vi "Main.vi"(11 "Module Admin":refnum<class "Delacor_lib_QMH_Module Admin.lvclass">) -> ()   [LabVIEW 2023, in "Analog Input.lvlib"]
doc: "This template is based off of the Queued Message Handler design pattern and the Queued Message Handler project template that ships with LabVIEW.\n\nThe main difference is that the queue is private to this module and communication between modules is performed via Broadcast and Request events.\n\nRequest events are wrapped in public API methods and are handled in the Event Handling Loop (EHL) of this VI. Any module can register for Broadcast events sent by this module. The EHL generates messages based on user interface actions.\n\nThe Message Handling Loop (MHL) processes messages generated by the EHL, or by other messages. The messages are string values, so new messages can be added easily to the Message Cases case structure in the MHL. Each message cluster can also provide an optional value for Message Data, which is a variant that can be converted to whatever message-specific data is required.\n_____\nBased on DQMH Dev Tools: Project Template 7.1.1.1528."
uses:
  Analog Input.lvlib
  <vilib>/Delacor/Delacor QMH/Libraries/Module Admin_class/Delacor_lib_QMH_Module Admin.lvclass
  Module Data--cluster.ctl
  <vilib>/myRIO/Instrument Drivers/Onboard IO/AI/typedefs/AI Reference.ctl
  <vilib>/myRIO/Common/Instrument Driver Framework/Utilities/typedefs/myRIO Generic Hardware Reference.ctl
  <vilib>/myRIO/Common/Instrument Driver Framework/Utilities/typedefs/Hardware Version Enum.ctl
  <vilib>/myRIO/Common/Instrument Driver Framework/Utilities/typedefs/myRIO v1.0 Reference.ctl
  <vilib>/myRIO/Common/Instrument Driver Framework/Utilities/typedefs/Generic FPGA Reference.ctl
  <vilib>/myRIO/Common/Instrument Driver Framework/myRIO v1.0/AI/typedefs/AI Channels List.ctl
  <vilib>/myRIO/Common/Instrument Driver Framework/myRIO v1.0/AI/typedefs/AI Channels Enum.ctl
  <vilib>/myRIO/Common/Instrument Driver Framework/Utilities/typedefs/Analog Scaling Constants List.ctl
  <vilib>/myRIO/Common/Instrument Driver Framework/Utilities/typedefs/Analog Scaling Constants.ctl
  Stop Argument--cluster.ctl
  <vilib>/Delacor/Delacor QMH/Libraries/Message Queue_class/Delacor_lib_QMH_Message Queue.lvclass/Delacor_lib_QMH_Message Queue.ctl
  <vilib>/Delacor/Delacor QMH/Libraries/Module Admin_class/Delacor_lib_QMH_Module Admin.lvclass/Delacor_lib_QMH_Module Admin.ctl
  <vilib>/userDefined/High Color/nirio_resource_hc.ctl
  <vilib>/Delacor/Delacor QMH/Libraries/Message Queue_class/Delacor_lib_QMH_Enqueue Message (Single).vi
  <vilib>/Delacor/Delacor QMH/Libraries/Module Admin_class/Delacor_lib_QMH_Get External Launch.vi
  <vilib>/myRIO/Common/Instrument Driver Framework/myRIO v1.0/AI/vis/myRIO v1.1 Open AI.vi
  <vilib>/myRIO/Common/Instrument Driver Framework/Utilities/vis/Validate Channels.vi
  <vilib>/myRIO/Common/Instrument Driver Framework/myRIO v1.0/AI/vis/myRIO v1.0 Reserve AI.vi
  <vilib>/myRIO/Common/Instrument Driver Framework/myRIO v1.0/AI/vis/myRIO v1.0 Close AI.vi
  <vilib>/myRIO/Common/Instrument Driver Framework/myRIO v1.0/AI/vis/myRIO v1.0 Build MUX Configuration AI.vi
  <vilib>/myRIO/Common/Instrument Driver Framework/myRIO v1.0/Resource Manager/vis/myRIO v1.0 Reserve Channel List.vi
  <vilib>/myRIO/Common/Instrument Driver Framework/myRIO v1.0/AI/vis/myRIO v1.0 Unreserve AI.vi
  <vilib>/myRIO/Common/Instrument Driver Framework/myRIO v1.0/Resource Manager/vis/myRIO v1.0 Reserve Channel.vi
  <vilib>/myRIO/Common/Instrument Driver Framework/myRIO v1.0/Resource Manager/vis/myRIO v1.0 Unreserve Channel.vi
  <vilib>/myRIO/Common/Instrument Driver Framework/myRIO v1.0/Resource Manager/vis/myRIO v1.0 Unreserve Channel List.vi
  <vilib>/myRIO/Common/Instrument Driver Framework/myRIO v1.0/Resource Manager/vis/myRIO v1.0 Build Mutex Name.vi
  <vilib>/Utility/VariantDataType/GetNumericInfo.vi
  <vilib>/myRIO/Common/Instrument Driver Framework/myRIO v1.0/myRIO v1.1 Open.vi
  <vilib>/myRIO/Common/Instrument Driver Framework/myRIO v1.0/AI/vis/myRIO v1.0 Get Scaling Constants AI.vi
  <vilib>/myRIO/Common/Instrument Driver Framework/Utilities/vis/IO Manager.vi
  <vilib>/myRIO/Common/Instrument Driver Framework/Utilities/vis/Configuration Manager.vi
  <vilib>/myRIO/Common/Instrument Driver Framework/myRIO v1.0/myRIO v1.0 Close.vi
  <vilib>/myRIO/Common/Instrument Driver Framework/myRIO v1.0/AI/vis/myRIO v1.0 Read AI.vi
  <vilib>/myRIO/Instrument Drivers/Onboard IO/AI/vis/myRIO AI Open.xnode
  <vilib>/Delacor/Delacor QMH/Libraries/Message Queue_class/Delacor_lib_QMH_Message Queue.lvclass
  <vilib>/myRIO/Instrument Drivers/Onboard IO/AI/AI.lvlib
panel:
  out "error out":errorcluster
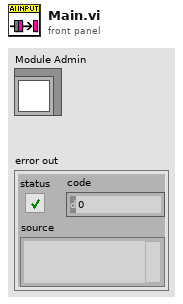
[diagram p1: front panel]
types:
  T1 = typedef "Analog Input.lvlib/Request Events--cluster.ctl" = cluster{"Stop Module":refnum<user-event>, "Show Panel":refnum<user-event>, "Hide Panel":refnum<user-event>, "Get Module Execution Status":refnum<user-event>, "Show Diagram":refnum<user-event>, "Private.Open Connection":refnum<user-event>, "Read Analog":refnum<user-event>}
  T2 = typedef "Analog Input.lvlib/Module Data--cluster.ctl" = cluster{"Status":string, "AI Reference":T3}
  T3 = typedef "AI.lvlib/AI Reference.ctl" = cluster{"myRIO Reference":T4, "AI Channels List":T8, "AI Scaling Constants List":T10}
  T4 = typedef "myRIO Generic Hardware Reference.ctl" = cluster{"myRIO Model":T5, "myRIO Hardware Reference":T6}
  T5 = typedef "Hardware Version Enum.ctl" = enum16{"Unknown", "myRIO-1900", "myRIO-1950", "roboRIO", "NI ELVIS RIO CM", "ELVIS III"}
  T6 = typedef "myRIO v1.0 Reference.ctl" = cluster{"Generic FPGA Reference":T7, "Allow multiple opens":bool}
  T7 = typedef "Generic FPGA Reference.ctl" = refnum<k20>
  T8 = typedef "AI Channels List.ctl" = T9[]
  T9 = typedef "AI Channels Enum.ctl" = enum16{"Not Connected", "AudioIn/Left", "AudioIn/Right", "C/AI0", "C/AI1", "A/AI0", "A/AI1", "A/AI2", "A/AI3", "A/AI4", "A/AI5", "A/AI6", "A/AI7", "B/AI0", "B/AI1", "B/AI2", "B/AI3", "B/AI4", "B/AI5", "B/AI6", "B/AI7", "AI/AI0", "AI/AI1", "AI/AI2", "AI/AI3", "A/AI0 (DIFF)", "A/AI1 (DIFF)", "A/AI2 (DIFF)", "A/AI3 (DIFF)", "B/AI0 (DIFF)", "B/AI1 (DIFF)", "B/AI2 (DIFF)", "B/AI3 (DIFF)"}
  T10 = typedef "Analog Scaling Constants List.ctl" = T11[]
  T11 = typedef "Analog Scaling Constants.ctl" = cluster{"LSB Weight (Volts)":dbl, "Offset (Volts)":dbl, "Signed?":bool}
  T12 = enum32{"invalid lock state", "Not Locked", "Locked (No Password)", "Password-protected"}
  T13 = typedef "Analog Input.lvlib/Stop Argument--cluster.ctl" = cluster{"Origin":string, "Exit via Stop Module Req?":bool, "Wait for Module to stop?":bool}
  T14 = typedef "nirio_resource_hc.ctl" = tag
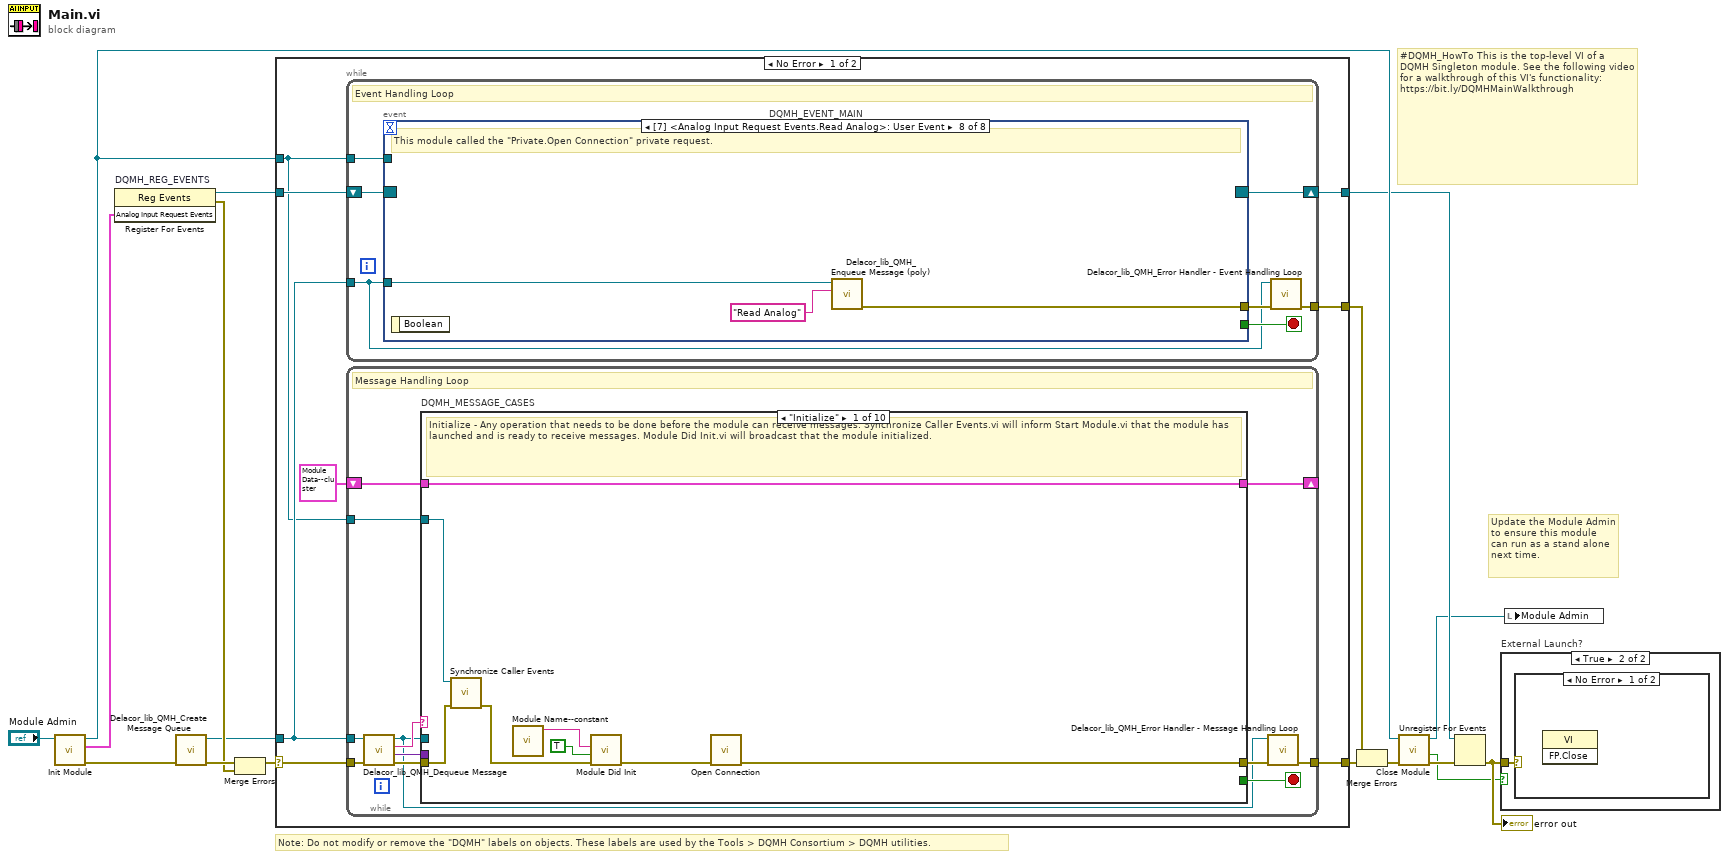
[diagram p0: block diagram]
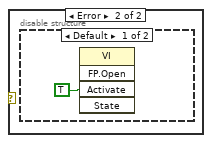
[diagram p3: hidden frame]
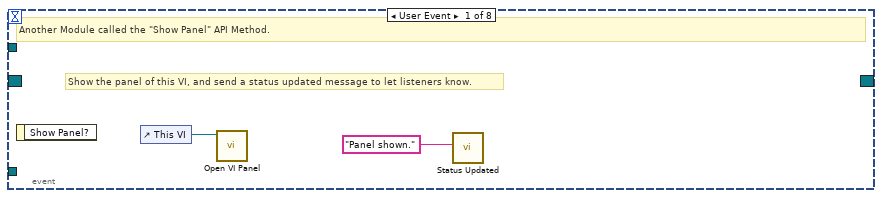
[diagram p5: hidden frame]
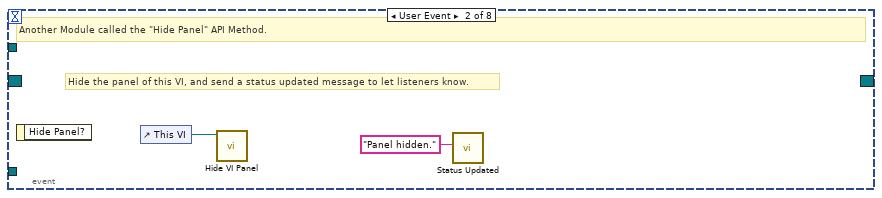
[diagram p6: hidden frame]
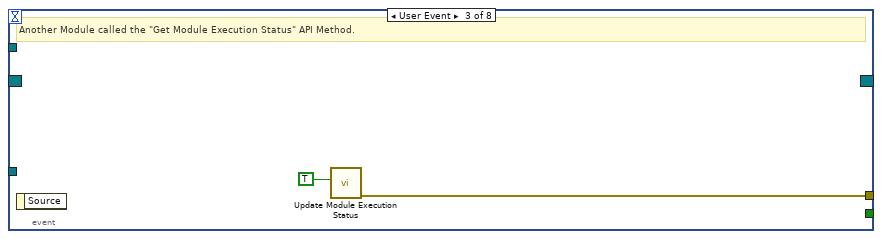
[diagram p7: hidden frame]
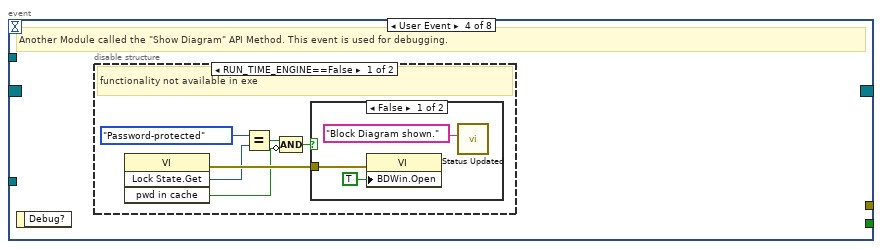
[diagram p8: hidden frame]
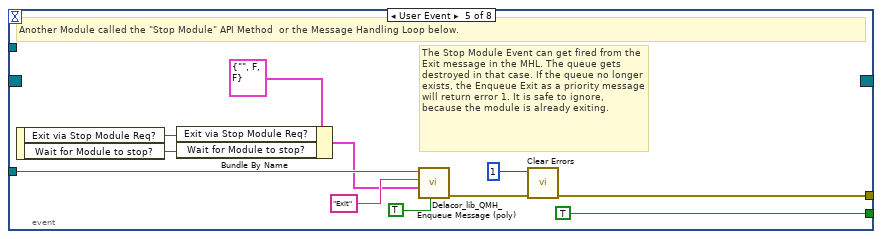
[diagram p11: hidden frame]
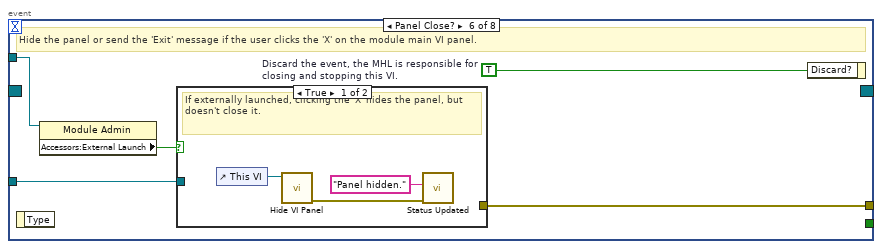
[diagram p12: hidden frame]
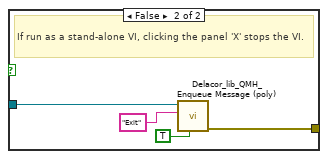
[diagram p13: hidden frame]
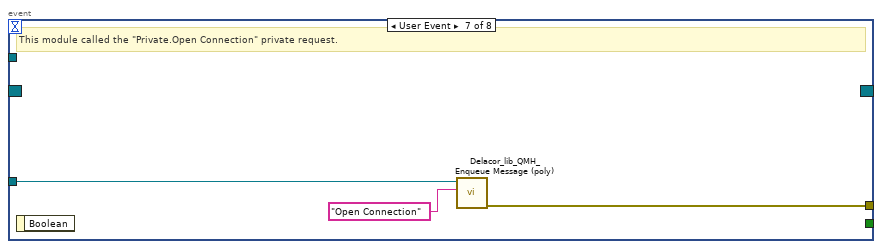
[diagram p14: hidden frame]
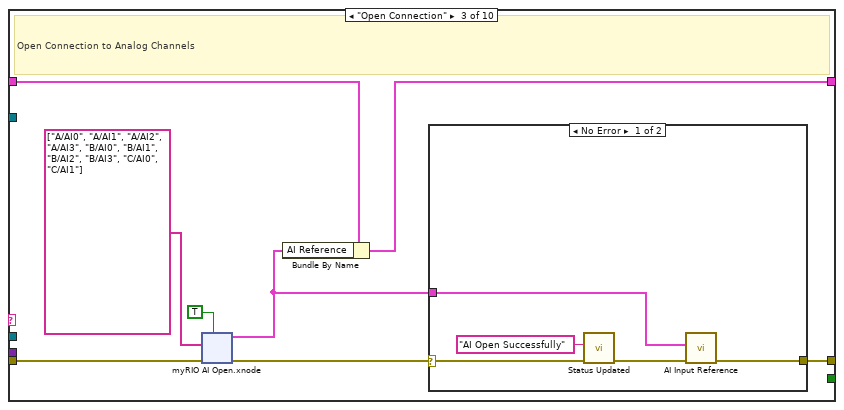
[diagram p16: hidden frame]
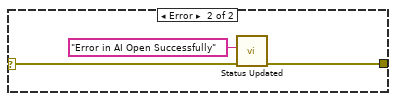
[diagram p17: hidden frame]
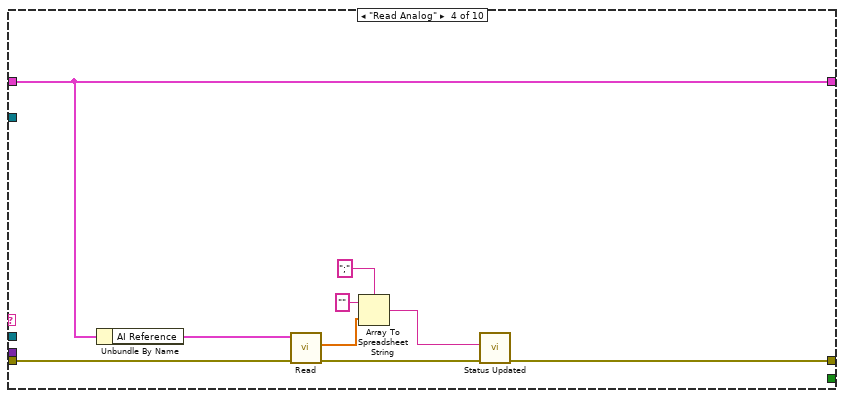
[diagram p18: hidden frame]
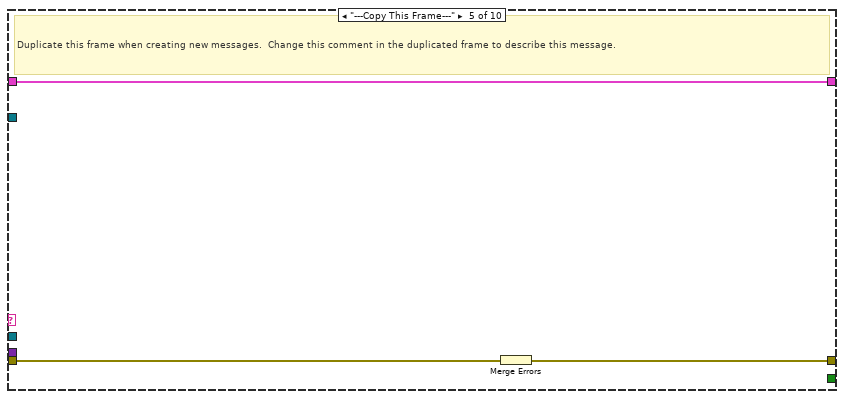
[diagram p19: hidden frame]
diagram:
  # "#DQMH_HowTo This is the top-level VI of a DQMH Singleton module. See the following video for a walkthrough of this VI's functionality: https://bit.ly/DQMHMainWalkthrough"
  # "Note: Do not modify or remove the \"DQMH\" labels on objects. These labels are used by the Tools > DQMH Consortium > DQMH utilities."
  # "Update the Module Admin to ensure this module can run as a stand alone next time."
  n1 = call "Init Module.vi"("Singleton Module Admin in"="Module Admin") -> ("error out"=w16:errorcluster, "Analog Input Request Events"=w5:T1, "Singleton Module Admin out"=w8:refnum<class "Delacor_lib_QMH_Module Admin.lvclass">)  [unwired: 8 in]
  n2 = register-events "DQMH_REG_EVENTS"(w5) -> (reference out=w6:refnum<event-registration>, error out=w9:errorcluster)  [unwired: 2 in]
  n3 = call <vilib>:"Delacor_lib_QMH_Create Message Queue.vi"("error in"=w16) -> ("error out"=w11:errorcluster, "Message Queue"=w4:refnum<class "Delacor_lib_QMH_Message Queue.lvclass">)  [unwired: 9 in]
  n4 = Merge Errors(w11, w9) -> (w10:errorcluster)
  n5 = case shown="No Error" w10 {
    selector: w10 -> [w23 w206]
    tunnel: [w25 w205] -> w17
    tunnel: [w22 w204] -> w7
    tunnel: w6 -> [w20 w204]
    tunnel: w4 -> [w19 w199]
    tunnel: [w24 _] -> w14
    tunnel: w8 -> [w18 w200]
    frame No Error {
      n6 = while {
        tunnel: w19 -> [w26]
        shift-right: [w29] -> w22
        shift-left: w20 -> [w30]
        tunnel: [w31] -> w24
        tunnel: w18 -> [w27]
        stop <- w28 stop-if-true
        # "Event Handling Loop"
        n7 = event "DQMH_EVENT_MAIN" shown="[7] <Analog Input Request Events.Read Analog>: User Event" {
          selector: w30 -> [_ _ _ _ _ _ _ _]
          dyn-events: [_ _ _ _ _ _ _ _] -> w29
          timeout: _ -> [_ _ _ _ _ _ _ _]
          tunnel: [_ _ _ _ TRUE ("Discard?") _ _ _] -> w28
          tunnel: w26 -> [_ _ _ _ w54 w61 w73 w76]
          tunnel: [_ _ w38 _ w57 w63 w71 w74] -> w32
          tunnel: w27 -> [_ _ _ _ _ w60 _ _]
          event User Event {
            # "Show the panel of this VI, and send a status updated message to let listeners know."
            # "Another Module called the \"Show Panel\" API Method."
            n8 = event-data() -> ()  [unwired: 1 in, 1 out]
            n9 = control-ref of="This VI"() -> (w34:refnum<vi>)
            n10 = call "Open VI Panel.vi"("VI"=w34) -> ()  [unwired: 10 in, 1 out]
            n11 = call "Status Updated.vi"("Status"="Panel shown." ("format string")) -> ()  [unwired: 10 in, 1 out]
          }
          event User Event {
            # "Hide the panel of this VI, and send a status updated message to let listeners know."
            # "Another Module called the \"Hide Panel\" API Method."
            n12 = event-data() -> ()  [unwired: 1 in, 1 out]
            n13 = control-ref of="This VI"() -> (w36:refnum<vi>)
            n14 = call "Hide VI Panel.vi"("VI"=w36) -> ()  [unwired: 10 in, 1 out]
            n15 = call "Status Updated.vi"("Status"="Panel hidden." ("format string")) -> ()  [unwired: 10 in, 1 out]
          }
          event User Event {
            # "Another Module called the \"Get Module Execution Status\" API Method."
            n16 = event-data() -> ()  [unwired: 1 in, 1 out]
            n17 = call "Update Module Execution Status.vi"("Running?"=TRUE) -> ("error out"=w38:errorcluster)  [unwired: 10 in]
          }
          event User Event {
            # "Another Module called the \"Show Diagram\" API Method. This event is used for debugging."
            n18 = event-data() -> ()  [unwired: 1 in, 1 out]
            n19 = disable-structure shown="RUN_TIME_ENGINE==False" {
              frame condition #0 (active) {
                # "functionality not available in exe"
                n20 = invoke on="Invoke Node" class="VI" method="Lock State.Get"() -> (error out=w44:errorcluster, "Get Lock State"=w43:T12, "pwd in cache"=w40:bool)  [unwired: 4 in, 1 out]
                n21 = Equal?(x=T12."Password-protected", y=w43) -> (x = y?=w41:bool)
                n22 = Compound Arithmetic op=AND(w41, invert w40) -> (w39:bool)
                n23 = case shown="False" w39 {
                  tunnel: w44 -> [w47 _]
                  frame False {
                    n24 = property on="Property Node" class="VI"(error in=w47, "BDWin.Open"=TRUE ("Block Diagram Window:Open")) -> ()  [unwired: 1 in, 2 out]
                    n25 = call "Status Updated.vi"("Status"="Block Diagram shown." ("format string")) -> ()  [unwired: 10 in, 1 out]
                  }
                  frame True {
                    # "Password-protected VI, and the password is not in the cache. Do not show the diagram."
                  }
                }
              }
              frame condition #1 {
              }
            }
          }
          event User Event {
            # "The Stop Module Event can get fired from the Exit message in the MHL. The queue gets destroyed in that case. If the queue no longer exists, the Enqueue Exit as a priority message will return error 1. It is safe to ignore, because the module is already exiting."
            # "Another Module called the \"Stop Module\" API Method  or the Message Handling Loop below."
            n26 = event-data() -> ("Exit via Stop Module Req?"=w50:bool, "Wait for Module to stop?"=w49:bool)  [unwired: 1 in]
            n27 = Bundle By Name(cluster=T13 {"Origin"="", "Exit via Stop Module Req?"=FALSE, "Wait for Module to stop?"=FALSE} ("Stop Argument"), "Exit via Stop Module Req?"=w50, "Wait for Module to stop?"=w49) -> (w48:T13)
            n28 = call-poly <vilib>:"Delacor_lib_QMH_Enqueue Message (poly).vi"("Priority Message? (F)"=TRUE, "Message Data"=w48, "Message"="Exit", "Message Queue in"=w54) -> ("error out"=w58:errorcluster)  [unwired: 6 in, 1 out]
            n29 = call <vilib>:"Clear Errors.vi"("error in (no error)"=w58, "specific error code to clear (0: all)"=1) -> ("error out"=w57:errorcluster)  [unwired: 4 in, 1 out]
          }
          event Panel Close? {
            w62 = TRUE  # Discard the event, the MHL is responsible for closing and stopping this VI.
            # "Hide the panel or send the 'Exit' message if the user clicks the 'X' on the module main VI panel."
            n30 = event-data() -> ()  [unwired: 1 in, 1 out]
            n31 = property on="Property Node" class="Module Admin"(reference=w60) -> ("Accessors:External Launch"=w59:bool)  [unwired: 1 in, 2 out]
            n32 = case shown="True" w59 {
              tunnel: w61 -> [_ w69]
              tunnel: [_ w70] -> w63
              frame True {
                # "If externally launched, clicking the 'X' hides the panel, but doesn't close it."
                n33 = control-ref of="This VI"() -> (w66:refnum<vi>)
                n34 = call "Hide VI Panel.vi"("VI"=w66) -> ("error out"=w64:errorcluster)  [unwired: 10 in]
                n35 = call "Status Updated.vi"("error in"=w64, "Status"="Panel hidden." ("format string")) -> ()  [unwired: 9 in, 1 out]
              }
              frame False {
                # "If run as a stand-alone VI, clicking the panel 'X' stops the VI."
                n36 = call-poly <vilib>:"Delacor_lib_QMH_Enqueue Message (poly).vi"("Priority Message? (F)"=TRUE, "Message"="Exit", "Message Queue in"=w69) -> ("error out"=w70:errorcluster)  [unwired: 7 in, 1 out]
              }
            }
            n37 = event-data ("Event Filter Node")("Discard?"=w62) -> ()  [unwired: 1 in, 1 out]
          }
          event User Event {
            # "This module called the \"Private.Open Connection\" private request."
            n38 = event-data() -> ()  [unwired: 1 in, 1 out]
            n39 = call-poly <vilib>:"Delacor_lib_QMH_Enqueue Message (poly).vi"("Message"="Open Connection", "Message Queue in"=w73) -> ("error out"=w71:errorcluster)  [unwired: 8 in, 1 out]
          }
          event User Event {
            # "This module called the \"Private.Open Connection\" private request."
            n40 = event-data() -> ()  [unwired: 1 in, 1 out]
            n41 = call-poly <vilib>:"Delacor_lib_QMH_Enqueue Message (poly).vi"("Message"="Read Analog", "Message Queue in"=w76) -> ("error out"=w74:errorcluster)  [unwired: 8 in, 1 out]
          }
        }
        n42 = call-dynamic "Delacor_lib_QMH_Error Handler - Event Handling Loop.vi"("error in"=w32, "Message Queue in"=w26) -> ("dup error in"=w31:errorcluster)  [unwired: 8 in, 1 out]
      }
      n43 = while {
        tunnel: w19 -> [w77]
        shift-right: [w85] -> _
        shift-left: T2 {"Status"="", "AI Reference"={"myRIO Reference"={"myRIO Model"=enum."Unknown", "myRIO Hardware Reference"={"Generic FPGA Reference"=refnum, "Allow multiple opens"=FALSE}}, "AI Channels List"=[], "AI Scaling Constants List"=[]}} ("Data Cluster") -> [w86]
        tunnel: w23 -> [w88]
        tunnel: [w80] -> w25
        tunnel: w18 -> [w81]
        stop <- w84 stop-if-true
        # "Message Handling Loop"
        n44 = call-dynamic "Delacor_lib_QMH_Dequeue Message.vi"("error in"=w88, "Message Queue in"=w77) -> ("error out"=w87:errorcluster, "Message Data"=w82:variant, "Message"=w83:string, "Message Queue out"=w78:refnum<class "Delacor_lib_QMH_Message Queue.lvclass">)  [unwired: 6 in]
        n45 = case "DQMH_MESSAGE_CASES" shown="\"Initialize\"" w83 {
          selector: w83 -> [_ _ _ _ _ _ _ _ _ w194]
          tunnel: w78 -> [_ _ _ _ _ _ _ w159 w182 _]
          tunnel: w87 -> [w96 w98 w106 w141 w144 w146 w155 w166 w188 w197]
          tunnel: [w89 w98 w101 w134 w143 w146 w154 w162 w183 w198] -> w79
          tunnel: w86 -> [w93 w97 w103 w140 w142 w145 w152 w161 w174 w195]
          tunnel: [w93 w97 w104 w140 w142 w145 w152 w161 w174 w195] -> w85
          tunnel: [_ _ _ _ _ _ _ _ w181 _] -> w84
          tunnel: w82 -> [_ _ _ _ _ _ _ w160 w180 _]
          tunnel: w81 -> [w94 _ _ _ _ _ _ w158 w175 _]
          frame "Initialize" {
            # "Initialize - Any operation that needs to be done before the module can receive messages. Synchronize Caller Events.vi will inform Start Module.vi that the module has launched and is ready to receive messages. Module Did Init.vi will broadcast that the module initialized."
            n46 = call "Synchronize Caller Events.vi"("error in"=w96, "Singleton Module Admin in"=w94) -> ("error out"=w95:errorcluster)  [unwired: 8 in, 1 out]
            n47 = call "Module Name--constant.vi"() -> ("Module Name"=w91:string)  [unwired: 11 in]
            n48 = call "Module Did Init.vi"("error in"=w95, "Initialized?"=TRUE, "Origin"=w91) -> ("error out"=w90:errorcluster)  [unwired: 8 in]
            n49 = call "Open Connection.vi"("error in"=w90) -> ("error out"=w89:errorcluster)  [unwired: 10 in]
          }
          frame "---Module Specific---" {
            # "Separator -- The following cases handle messages specific to this Module."
          }
          frame "Open Connection" {
            # "Open Connection to Analog Channels"
            n50 = xnode "myRIO AI Open.xnode"("error in (no error)"=w106, "Allow multiple opens?"=TRUE, "Channel Names"=tag[] ["A/AI0", "A/AI1", "A/AI2", "A/AI3", "B/AI0", "B/AI1", "B/AI2", "B/AI3", "C/AI0", "C/AI1"]) -> ("error out"=w102:errorcluster, "AI Ref Out"=w100:T3)
            n51 = Bundle By Name(cluster=w103, "AI Reference"=w100) -> (w104:T2)
            n52 = case shown="No Error" w102 {
              selector: w102 -> [w111 w114]
              tunnel: [w108 w113] -> w101
              tunnel: w100 -> [w107 _]
              frame No Error {
                n53 = call "Status Updated.vi"("error in"=w111, "Status"="AI Open Successfully") -> ("error out"=w109:errorcluster)  [unwired: 9 in]
                n54 = call "AI Input Reference.vi"("error in"=w109, "AI Reference"=w107) -> ("error out"=w108:errorcluster)  [unwired: 9 in]
              }
              frame Error {
                n55 = call "Status Updated.vi"("error in"=w114, "Status"="Error in AI Open Successfully") -> ("error out"=w113:errorcluster)  [unwired: 9 in]
              }
            }
          }
          frame "Read Analog" {
            n56 = Unbundle By Name(w140) -> ("AI Reference"=w139:T3)
            n57 = call <vilib>:"Read.vi"("error in (no error)"=w141, "AI Ref In"=w139) -> ("error out"=w136:errorcluster, "Values"=w138:dbl[])  [unwired: 7 in, 1 out]
            n58 = Array To Spreadsheet String(delimiter (Tab)=";", array=w138, 3:"" ("format string")) -> (spreadsheet string=w135:string)
            n59 = call "Status Updated.vi"("error in"=w136, "Status"=w135) -> ("error out"=w134:errorcluster)  [unwired: 9 in]
          }
          frame "---Copy This Frame---" {
            # "Duplicate this frame when creating new messages.  Change this comment in the duplicated frame to describe this message."
            n60 = Merge Errors(w144) -> (w143:errorcluster)
          }
          frame "---Exit and Error Handling---" {
            # "Separator - The following cases handle errors and exit messages."
          }
          frame "Simulate MHL Error" {
            # "#DQMH_HowTo The 'Simulate MHL Error' button  illustrates how the MHL handles errors. This event is instructional in nature and can be removed."
            # "Simulate an error occurring at the MHL"
            n61 = call "Module Name--constant.vi"() -> ("Module Name"=w148:string)  [unwired: 11 in]
            n62 = Format Into String(format string="Simulated error originating at Message Handling Loop in %s", w148) -> (resulting string=w149:string)  [unwired: 2 in, 1 out]
            n63 = call <vilib>:"Error Cluster From Error Code.vi"("show call chain? (False)"=TRUE, "error message (\"\")"=w149, "error code (0)"=5001) -> ("error out"=w153:errorcluster)  [unwired: 6 in]
            n64 = Merge Errors(w155, w153) -> (w154:errorcluster)
          }
          frame "Error" {
            # "#DQMH_CodeRecommended - If the module is running in standalone mode (External Launch = FALSE), this code will pop up an error dialog and call the 'Exit' message if an error occurs. Add more fine-grained error management here."
            # "Error - Check the error message data and respond accordingly. This message is sent by the \"Error Handler\" VIs at the end of each loop in this application."
            n65 = property on="Property Node" class="Module Admin"(reference=w158) -> ("Accessors:External Launch"=w157:bool)  [unwired: 1 in, 2 out]
            n66 = Variant To Data(error in=w166, type=errorcluster {"status"=FALSE, "code"=0, "source"=""} ("error constant"), Variant=w160) -> (data=w156:errorcluster, error out=w164:errorcluster)
            n67 = local write "error out"(w156) -> ()
            n68 = call "Error Reported.vi"("Error"=w156) -> ()  [unwired: 10 in, 1 out]
            n69 = case shown="False" w157 {
              tunnel: [w171 _] -> w163
              tunnel: w159 -> [w169 _]
              tunnel: w156 -> [w170 _]
              frame False {
                n70 = disable-structure shown="Default" {
                  disable-tunnel: w170 -> [w172 _]
                  frame condition #0 (active) {
                    # "If the module is running standalone, then pop up an error dialog and call the \"Exit\" message."
                    n71 = call <vilib>:"Simple Error Handler.vi"("error in (no error)"=w172) -> ()  [unwired: 4 in, 5 out]
                  }
                  frame condition #1 {
                    # "To prevent the Simple Error Handler VI from being loaded (e.g. when deploying to a Real-Time target), add the Conditional Disable Symbol \"DQMH_Disable_SEH\" to your project and set it to TRUE."
                  }
                }
                n72 = call-poly <vilib>:"Delacor_lib_QMH_Enqueue Message (poly).vi"("Priority Message? (F)"=TRUE, "Message"="Exit", "Message Queue in"=w169) -> ("error out"=w171:errorcluster)  [unwired: 7 in, 1 out]
              }
              frame True {
                # "If the module was launched externally, calling the Error Reported broadcast VI is the only action performed by the \"Error\" message. The module's caller can then process the error appropriately."
              }
            }
            n73 = Merge Errors(w164, w163) -> (w162:errorcluster)
          }
          frame "Exit" {
            w179 = 91  # 91: not all Exit messages will have an argument
            w181 = TRUE  # Stop the VI
            # "Release the message queue reference"
            # "Exit - Exit the application."
            n74 = Variant To Data(error in=w188, type=T13 {"Origin"="", "Exit via Stop Module Req?"=FALSE, "Wait for Module to stop?"=FALSE} ("Stop Argument"), Variant=w180) -> (data=w177:T13, error out=w185:errorcluster)
            n75 = call <vilib>:"Clear Errors.vi"("error in (no error)"=w185, "specific error code to clear (0: all)"=w179) -> ("error out"=w187:errorcluster)  [unwired: 4 in, 1 out]
            n76 = control-ref of="This VI"() -> (w176:refnum<vi>)
            n77 = call-dynamic "Delacor_lib_QMH_Release Message Queue.vi"("error in"=w187, "Message Queue"=w182) -> ("error out"=w186:errorcluster)  [unwired: 9 in]
            n78 = call "Handle Exit.vi"("Stop Argument"=w177, "Admin in"=w175, "VI reference"=w176) -> ("error out"=w184:errorcluster)  [unwired: 7 in, 1 out]
            n79 = Merge Errors(w186, w184) -> (w183:errorcluster)
            n80 = Unbundle By Name(w174) -> ("AI Reference"=w173:T3)
            n81 = call "Error Reported.vi"("Error"=w183) -> ()  [unwired: 10 in, 1 out]
            n82 = call <vilib>:"Close.vi"("AI Ref In"=w173) -> ()  [unwired: 10 in, 1 out]
          }
          frame Default {
            # "'Default' case only runs if there is a message that isn't defined in any of the other cases.  Output a programming error."
            n83 = call "Module Name--constant.vi"() -> ("Module Name"=w193:string)  [unwired: 11 in]
            n84 = Format Into String(format string="The invalid message string \"%s\" was received in the Message Handling Loop for module \"%s\".", w194, w193) -> (resulting string=w189:string)  [unwired: 2 in, 1 out]
            n85 = call <vilib>:"Error Cluster From Error Code.vi"("show call chain? (False)"=TRUE, "error message (\"\")"=w189, "error code (0)"=1) -> ("error out"=w196:errorcluster)  [unwired: 6 in]
            n86 = Merge Errors(w197, w196) -> (w198:errorcluster)
          }
        }
        n87 = call-dynamic "Delacor_lib_QMH_Error Handler - Message Handling Loop.vi"("error in"=w79, "Message Queue in"=w78) -> ("dup error in"=w80:errorcluster)  [unwired: 8 in, 1 out]
      }
    }
    frame Error {
      # "Synchronize Caller Events.vi will inform Start Module.vi that the module has launched and will let the code calling Start Module.vi register for broadcasts and would permit the caller receive the broadcast that an error occurred at launch time."
      n88 = call-dynamic "Delacor_lib_QMH_Release Message Queue.vi"("error in"=w206, "Message Queue"=w199) -> ("error out"=w205:errorcluster)  [unwired: 9 in]
      n89 = call "Synchronize Caller Events.vi"("Singleton Module Admin in"=w200) -> ("error out"=w207:errorcluster)  [unwired: 9 in, 1 out]
      n90 = call "Module Name--constant.vi"() -> ("Module Name"=w203:string)  [unwired: 11 in]
      n91 = Format Into String(format string="An error occurred during initialization. %s is no longer running.", w203) -> (resulting string=w201:string)  [unwired: 2 in, 1 out]
      n92 = Merge Errors(w205, w207) -> (w208:errorcluster)
      n93 = call "Error Reported.vi"("Additional Information"=w201, "Error"=w208) -> ()  [unwired: 9 in, 1 out]
    }
  }
  n94 = Merge Errors(w14, w17) -> (w13:errorcluster)
  n95 = call "Close Module.vi"("error in"=w13, "Module Admin in"=w8) -> ("error out"=w15:errorcluster, "External Launch"=w1:bool, "Module Admin out"=w2:refnum<class "Delacor_lib_QMH_Module Admin.lvclass">)  [unwired: 7 in]
  n96 = Unregister For Events(event registration refnum=w7, error in=w15) -> (error out=w12:errorcluster)
  "error out" <- w12
  n97 = case "External Launch?" shown="True" w1 {
    tunnel: w12 -> [_ w209]
    frame False {
    }
    frame True {
      n98 = case shown="No Error" w209 {
        frame No Error {
          n99 = invoke on="Invoke Node" class="VI" method="FP.Close"() -> ()  [unwired: 3 in, 3 out]
        }
        frame Error {
          n100 = disable-structure shown="Default" {
            frame condition #0 (active) {
              n101 = invoke class="VI" method="FP.Open"("Activate"=TRUE ("Activate?")) -> ()  [unwired: 4 in, 5 out]
            }
            frame condition #1 {
              # "Don't show panel on error if running inside a built EXE."
            }
          }
        }
      }
    }
  }
  n102 = local write "Module Admin"(w2) -> ()
